vi "VI Tree.vi"   [LabVIEW 2016, in "Tektronix AFG 1000 Series.lvlib"]
doc: "This is the instrument driver for the <B>Tektronix AFG 1000 Series</B>. The VI Tree displays all the user-callable VIs of the instrument driver in an organized table."
uses:
  Tektronix AFG 1000 Series.lvlib
  Configure/Configure Modulation (AM).vi
panel:
  # "(c) 2016 National Instruments.  ALL RIGHTS RESERVED."
  # "SEE DIAGRAM\nFOR VI TREE."
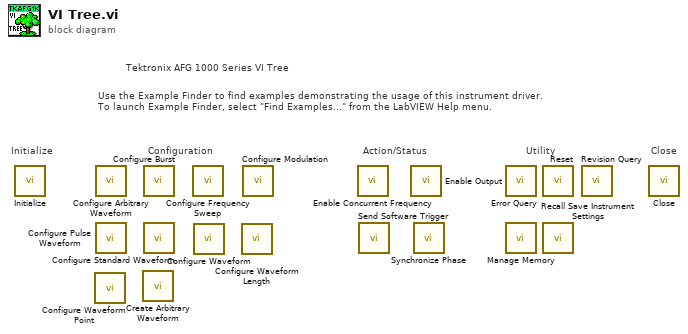
[diagram p0: block diagram]
diagram:
  # "Tektronix AFG 1000 Series VI Tree"
  # "Use the Example Finder to find examples demonstrating the usage of this instrument driver.\nTo launch Example Finder, select \"Find Examples...\" from the LabVIEW Help menu."
  # "Configuration"
  # "Utility"
  # "Action/Status"
  # "Close"
  # "Initialize"
  n1 = call "Initialize.vi"() -> ()  [unwired: 10 in, 2 out]
  n2 = call "Configure Waveform Point.vi"() -> ()  [unwired: 10 in, 2 out]
  n3 = call "Configure Arbitrary Waveform.vi"() -> ()  [unwired: 10 in, 2 out]
  n4 = call "Configure Pulse Waveform.vi"() -> ()  [unwired: 10 in, 2 out]
  n5 = call "Create Arbitrary Waveform.vi"() -> ()  [unwired: 10 in, 2 out]
  n6 = call "Configure Burst.vi"() -> ()  [unwired: 10 in, 2 out]
  n7 = call "Configure Standard Waveform.vi"() -> ()  [unwired: 10 in, 2 out]
  n8 = call "Configure Frequency Sweep.vi"() -> ()  [unwired: 10 in, 2 out]
  n9 = call "Configure Waveform.vi"() -> ()  [unwired: 10 in, 2 out]
  n10 = call "Configure Waveform Length.vi"() -> ()  [unwired: 10 in, 2 out]
  n11 = call-poly "Configure Modulation.vi"() -> ()  [unwired: 14 in, 2 out]
  n12 = call "Enable Concurrent Frequency.vi"() -> ()  [unwired: 10 in, 2 out]
  n13 = call "Send Software Trigger.vi"() -> ()  [unwired: 10 in, 2 out]
  n14 = call "Enable Output.vi"() -> ()  [unwired: 10 in, 2 out]
  n15 = call "Synchronize Phase.vi"() -> ()  [unwired: 10 in, 2 out]
  n16 = call "Error Query.vi"() -> ()  [unwired: 8 in, 4 out]
  n17 = call "Manage Memory.vi"() -> ()  [unwired: 9 in, 3 out]
  n18 = call "Reset.vi"() -> ()  [unwired: 10 in, 2 out]
  n19 = call "Recall Save Instrument Settings.vi"() -> ()  [unwired: 10 in, 2 out]
  n20 = call "Revision Query.vi"() -> ()  [unwired: 8 in, 4 out]
  n21 = call "Close.vi"() -> ()  [unwired: 11 in, 1 out]
